vi "Ping IP Address_O2.vi"(8 "error in":errorcluster, 9 "timeout (500 ms)":i32=500, 10 "count (1)":i32=1, 11 "host":string) -> (0 "error out":errorcluster, 2 "standard output":string, 3 "response?":bool)   [LabVIEW 2017]
doc: "Pings <B>host</B> count times with timeout and returns if there was a response."
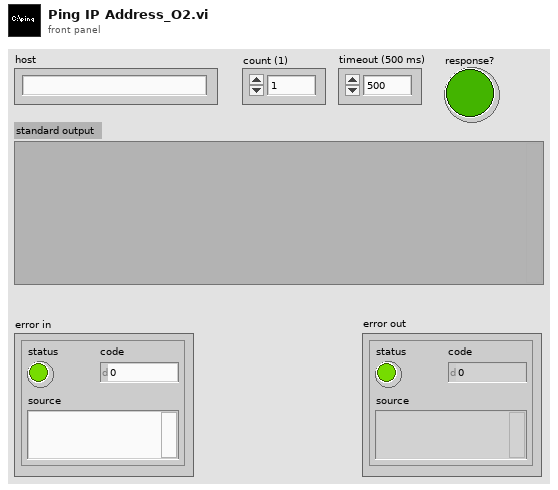
[diagram p1: front panel]
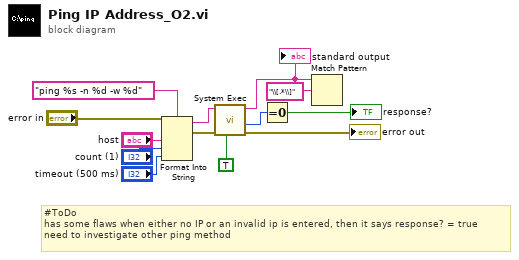
[diagram p0: block diagram]
diagram:
  # "#ToDo\nhas some flaws when either no IP or an invalid ip is entered, then it says response? = true\nneed to investigate other ping method"
  n1 = Format Into String(format string="ping %s -n %d -w %d", error in="error in", "host", "count (1)", "timeout (500 ms)") -> (resulting string=w11:string, error out=w12:errorcluster)  [unwired: 1 in]
  n2 = call <vilib>:"System Exec.vi"("run minimized? (F)"=TRUE, "error in (no error)"=w12, "command line"=w11) -> ("error out"=→"error out":errorcluster, "return code"=w9:i32, "standard output"=w6:string)  [unwired: 5 in, 1 out]
  "standard output" <- w6
  n3 = Equal To 0?(x=w9) -> (x = 0?=→"response?":bool)
  n4 = Match Pattern(string=w6, regular expression="\\[.*\\]") -> ()  [unwired: 1 in, 4 out]
